vi "WPI_SolenoidSet.vi"   [LabVIEW 2017]
doc: "Specifies whether the NI 9472 sends a 12 V signal to the solenoid you specify. When the solenoid receives the 12 V signal, the solenoid releases air, thus moving the associated robot part.\n\nThis software is licensed. Open the labview\\readme\\WPI Robotics Library Open Source License.txt file for more information."
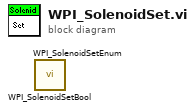
[diagram p0: block diagram]
diagram:
  n1 = call <vilib>:"WPI_SolenoidSetBool.vi"() -> ()  [unwired: 10 in, 2 out]
  n2 = call <vilib>:"WPI_SolenoidSetEnum.vi"() -> ()  [unwired: 10 in, 2 out]
